vi "GenesysPS.constructor.vi"(0 "name":string, 2 "data in":string, 5 "error in (no error)":errorcluster) -> (14 "i ref out":refnum<vi>, 16 "data out":string, 19 "error out":errorcluster)   [LabVIEW 2014, in "GenesysPS.lvlib"]
doc: "This is the constructor of a class.\n\nLicense Agreement for this software:\n\nCopyright (C)\nGesellschaft für Schwerionenforschung, GSI\nPlanckstr. 1\n64291 Darmstadt\nGermany\n\nContact: D.Beck@gsi.de \n\nThis program is free software; you can redistribute it and/or modify it under the terms of the GNU General Public License as published by the Free Software Foundation; either version 2 of the license, or (at your option) any later version.\n\nThis program is distributed in the hope that it will be useful, but WITHOUT ANY WARRANTY; without even the implied warranty of MERCHANTABILITY or FITNESS FOR A PARTICULAR PURPOSE. See the GNU General License for more details (http://www.gnu.org).\n\nGesellschaft für Schwerionenforschung, GSI\nPlanckstr. 1, 64291 Darmstadt, Germany\nFor all questions and ideas contact: M.Richter@gsi.de, H.Brand@gsi.de or D.Beck@gsi.de.\nLast update: 17-JUN-2004"
uses:
  GenesysPS.lvlib
  CSlibraries-extern/DimLVEvent/LVDimInterface/LVDimInterface.dim service type.ctl
  CSlibraries-extern/DimLVEvent/LVDimInterface/LVDimInterface.dic_info_service_queue.vi
  CS_Core/CSSystem/CSSystemLib/CSSystemLib.lvlib
  DIMPowerSupply/DIMPowerSupply.lvlib
  CS_Core/BaseProcess/BaseProcess.lvlib
  instr.lib/GENser/GENserDriver.lvlib
  CSlibraries-extern/DimLVEvent/LVDimInterface/LVDimInterface.lvlib
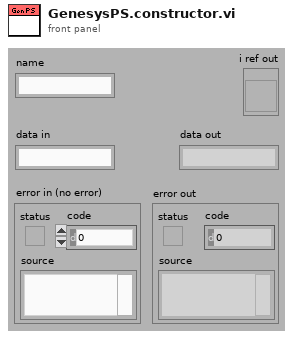
[diagram p1: front panel]
types:
  T1 = enum16{"SetAttribute", "GetAttribute", "CreateAttribute", "DestroyAttribute", "DestroyAllAtributes"}
  T2 = typedef "BaseProcess.lvlib/BaseProcess.i attribute.ctl" = cluster{"EventStatus":string, "EventError":i32, "PresetEvtWatchD":i32, "PresetPdcWatchD":i32, "EventTimeout":i32, "PeriodicInterval":i32, "Interface":string[], "Address":string[], "Special":string[], "PeriodicError":i32, "PeriodicStatus":string, "SuperProc":string, "Descriptors":T3[], "CaseRef":refnum<vi>, "PdcRef":refnum<vi>, "Thread Ref":refnum<vi>, "eventErrorID":i32, "eventStatusID":i32, "periodicErrorID":i32, "periodicStatusID":i32, "pdcCtrID":i32}
  T3 = typedef "BaseProcess.lvlib/BaseProcess.descriptor definition.ctl" = cluster{"selector":string, "descriptor":T4}
  T4 = typedef "BaseProcess.lvlib/BaseProcess.descriptor string definition.ctl" = string
  T5 = typedef "LVDimInterface.lvlib/LVDimInterface.dim service type.ctl" = u16
  T6 = typedef "GenesysPS.lvlib/GenesysPS.i attribute.ctl" = cluster{"VISA name/ Heizinger":refnum<visa-resource-name>, "GEN Addr":i32, "WithTempInt?":bool, "TempLimit":dbl, "TemperatureID":i32, "Temp queue":refnum<queue>}
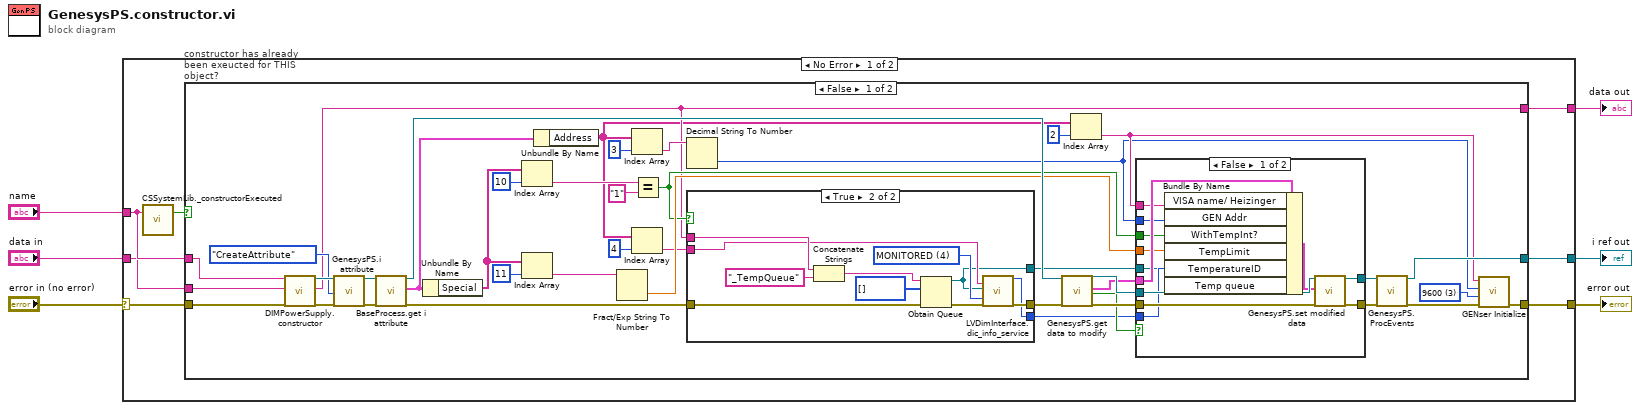
[diagram p0: block diagram]
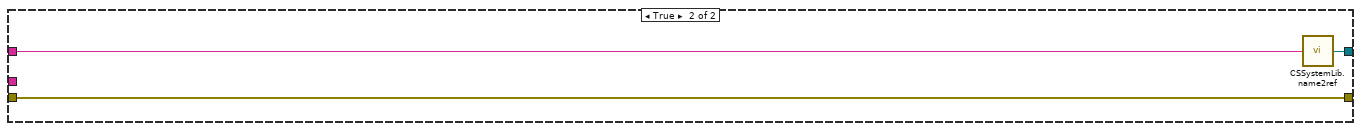
[diagram p4: hidden frame]
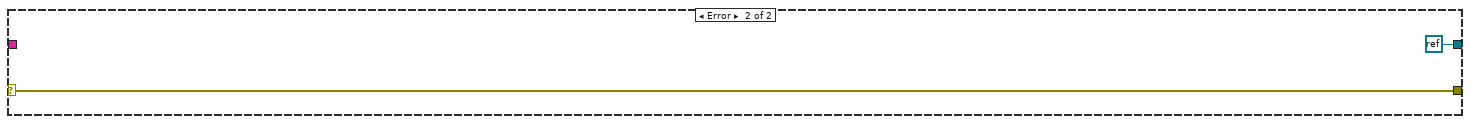
[diagram p5: hidden frame]
diagram:
  n1 = case shown="No Error" "error in (no error)" {
    selector: "error in (no error)" -> [w11 w84]
    tunnel: [w13 refnum<k0> refnum] -> w6
    tunnel: [w12 w84] -> w5
    tunnel: "name" -> [w9 _]
    tunnel: "data in" -> [w8 _]
    tunnel: [w7 _] -> w1
    frame No Error {
      n2 = call "CSSystemLib._constructorExecuted.vi"("name"=w9) -> ("constructor executed?"=w10:bool)  [unwired: 18 in]
      n3 = case "constructor has already been exeucted for THIS object?" shown="False" w10 {
        tunnel: [w37 w82] -> w13
        tunnel: [w35 w81] -> w12
        tunnel: w9 -> [w51 w83]
        tunnel: w11 -> [w50 w81]
        tunnel: w8 -> [w49 _]
        tunnel: [w19 _] -> w7
        frame False {
          w32 = u16 3 items=["1200", "2400", "4800", "9600", "19200"] ("BAUD")
          n4 = call "DIMPowerSupply.constructor.vi"("name"=w51, "data in"=w49, "error in (no error)"=w50) -> ("i ref out"=w54:refnum<vi>, "data out"=w19:string, "error out"=w53:errorcluster)  [unwired: 14 in]
          n5 = call "GenesysPS.i attribute.vi"("VI Refnum"=w54, "Action"=T1."CreateAttribute", "error in (no error)"=w53) -> ("VI Refnum out"=w46:refnum<vi>, "error out"=w44:errorcluster)  [unwired: 14 in, 1 out]
          n6 = call "BaseProcess.get i attribute.vi"("i ref in"=w46, "error in (no error)"=w44) -> ("i ref out"=w45:refnum<vi>, "i attribute"=w31:T2, "error out"=w21:errorcluster)  [unwired: 15 in]
          n7 = Unbundle By Name(w31) -> ("Special"=w30:string[])
          n8 = Index Array(array=w30, index=10) -> (element=w23:string)
          n9 = Index Array(array=w30, index=11) -> (element=w27:string)
          n10 = Unbundle By Name(w31) -> ("Address"=w18:string[])
          n11 = Fract/Exp String To Number(string=w27) -> (number=w26:dbl)  [unwired: 3 in, 1 out]
          n12 = Index Array(array=w18, index=3) -> (element=w42:string)
          n13 = Index Array(array=w18, index=4) -> (element=w16:string)
          n14 = Equal?(x=w23, y="1") -> (x = y?=w22:bool)
          n15 = Decimal String To Number(string=w42) -> (number=w33:i32)  [unwired: 2 in, 1 out]
          n16 = case shown="True" w22 {
            tunnel: w21 -> [w55 w64]
            tunnel: [w55 w66] -> w20
            tunnel: w19 -> [_ w60]
            tunnel: w16 -> [_ w59]
            tunnel: [_ w57] -> w15
            tunnel: [_ w56] -> w14
            frame False {
            }
            frame True {
              w58 = T5 4 items=["ONCE_ONLY"=1, "TIMED"=2, "MONITORED"=4] ("serviceType")
              n17 = Concatenate Strings(w60, "_TempQueue" ("string")) -> (w62:string)
              n18 = Obtain Queue(name (unnamed)=w62, element data type=i8[] [], error in (no error)=w64) -> (queue out=w56:refnum<queue>, error out=w63:errorcluster)  [unwired: 2 in, 1 out]
              n19 = call-poly "LVDimInterface.dic_info_service.vi"("serviceName"=w59, "queueRef"=w56, "serviceType"=w58, "error in (no error)"=w63) -> ("callBackID"=w57:i32, "error out"=w66:errorcluster)  [unwired: 14 in]
            }
          }
          n20 = call "GenesysPS.get data to modify.vi"("i ref in"=w45, "error in (no error)"=w20) -> ("i ref out"=w47:refnum<vi>, "i attribute"=w41:T6, "timed out"=w39:bool, "error out"=w48:errorcluster)  [unwired: 14 in]
          n21 = Index Array(array=w18, index=2) -> (element=w34:string)
          n22 = case shown="False" w39 {
            tunnel: w48 -> [w78 w79]
            tunnel: [w77 w79] -> w24
            tunnel: w47 -> [w76 w80]
            tunnel: [w75 w80] -> w38
            tunnel: w41 -> [w74 _]
            tunnel: w33 -> [w73 _]
            tunnel: w34 -> [w72 _]
            tunnel: w26 -> [w70 _]
            tunnel: w22 -> [w69 _]
            tunnel: w15 -> [w68 _]
            tunnel: w14 -> [w67 _]
            frame False {
              n23 = Bundle By Name(cluster=w74, "VISA name/ Heizinger"=w72, "GEN Addr"=w73, "WithTempInt?"=w69, "TempLimit"=w70, "TemperatureID"=w68, "Temp queue"=w67) -> (w71:T6)
              n24 = call "GenesysPS.set modified data.vi"("i ref in"=w76, "i attribute"=w71, "error in (no error)"=w78) -> ("i ref out"=w75:refnum<vi>, "error out"=w77:errorcluster)  [unwired: 15 in]
            }
            frame True {
            }
          }
          n25 = call "GenesysPS.ProcEvents.vi"("i ref in"=w38, "error in (no error)"=w24) -> ("i ref out"=w37:refnum<vi>, "error out"=w36:errorcluster)  [unwired: 16 in]
          n26 = call "GENser Initialize.vi"("error in (no error)"=w36, "BAUD"=w32, "GEN Addr"=w33, "VISA name"=w34) -> ("error out"=w35:errorcluster)  [unwired: 6 in, 1 out]
        }
        frame True {
          n27 = call "CSSystemLib.name2ref.vi"("name"=w83) -> ("obj refnum"=w82:refnum<vi>)
        }
      }
    }
    frame Error {
    }
  }
  "i ref out" <- w6
  "error out" <- w5
  "data out" <- w1
